vi "Flush.vi"(8 "error in (no error)":errorcluster, 11 "Queue in":refnum<class "Queue.lvclass">) -> (0 "error out":errorcluster, 2 "Remaining element":refnum<class "Data.lvclass">[](array[class]), 3 "Queue out":refnum<class "Queue.lvclass">)   [LabVIEW 2020, in "Data.lvlib" / "Queue.lvclass"]
doc: "Flush the queue."
uses:
  Queue.lvclass
  Data.lvclass
  Queue.lvclass/Queue.ctl
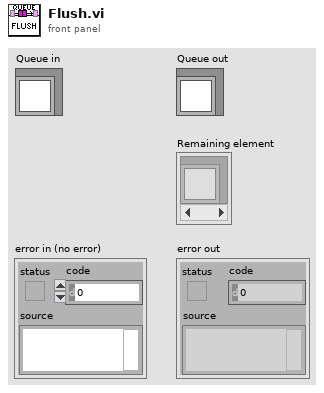
[diagram p1: front panel]
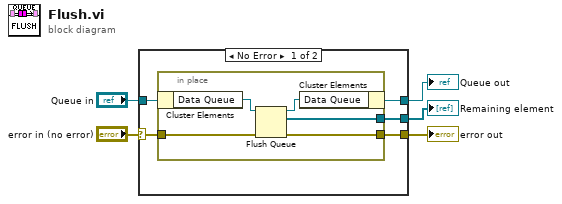
[diagram p0: block diagram]
diagram:
  n1 = case shown="No Error" "error in (no error)" {
    selector: "error in (no error)" -> [w8 w17]
    tunnel: [w7 w17] -> w4
    tunnel: [w9 w16] -> w2
    tunnel: "Queue in" -> [w10 w16]
    tunnel: [w6 _] -> w1
    frame No Error {
      n2 = in-place {
        in-place-border: w8 -> [w12]
        in-place-border: [w11] -> w7
        in-place-border: [w13] -> w6
        n3 = in-place-cluster #1(w10) -> ("Data Queue"=w15:refnum<queue>)
        n4 = Flush Queue(queue=w15, error in (no error)=w12) -> (queue out=w14:refnum<queue>, remaining elements=w13:refnum<class "Data.lvclass">[], error out=w11:errorcluster)
        n5 = in-place-cluster #1("Data Queue"=w14) -> (w9:refnum<class "Queue.lvclass">)
      }
    }
    frame Error {
    }
  }
  "error out" <- w4
  "Queue out" <- w2
  "Remaining element" <- w1
